vi "build.vi"(8 "error in (no error)":errorcluster, 10 "build_spec":T1, 11 "lv-build-default in":refnum<class "lv-builder.lvclass">) -> (0 "error out":errorcluster, 2 "[] generated_files":path[](array[path]), 3 "lv-build-default out":refnum<class "lv-builder.lvclass">)   [LabVIEW 2015, in "lv-builder.lvlib" / "lv-builder.lvclass"]
uses:
  lv-builder.lvclass
  lv-build/public/_controls/build_specification.ctl
  lv-build/public/_controls/build_type.ctl
  lv-builder.lvclass/lv-builder.ctl
  <vilib>/AppBuilder/AB_API_Simple/Set Build Specification Version (path).vi
  lv-builder.lvlib
  <vilib>/AppBuilder/AB_API_Simple/NI_App_Builder_API.lvlib
  lv-build/lv-build.lvlib
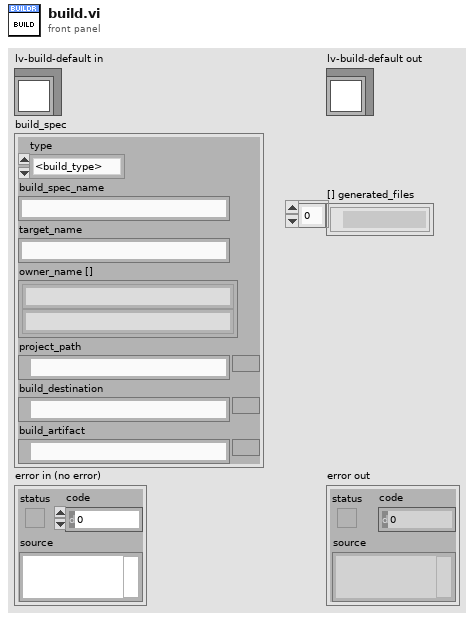
[diagram p1: front panel]
types:
  T1 = typedef "lv-build.lvlib/build_specification.ctl" = cluster{"type":T2, "build_spec_name":string, "target_name":string, "owner_name []":string[], "project_path":path, "build_destination":path, "build_artifact":path}
  T2 = typedef "lv-build.lvlib/build_type.ctl" = enum16{"<build_type>", "application_pc", "application_rt", "installer", "llb", "lvlibp", "zip", "fpga", "<null>"}
  T3 = typedef "NI_App_Builder_API.lvlib/Build Specification Version.ctl" = cluster{"Major":u16, "Minor":u16, "Fix":u16, "Build":u16}
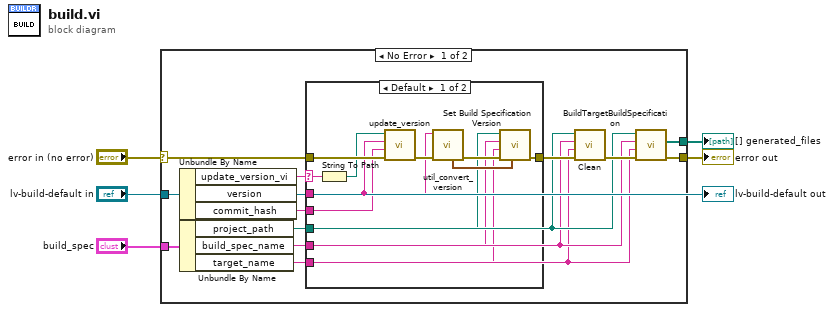
[diagram p0: block diagram]
diagram:
  n1 = case shown="No Error" "error in (no error)" {
    selector: "error in (no error)" -> [w16 w32]
    tunnel: [w10 w32] -> w3
    tunnel: "lv-build-default in" -> [w17 _]
    tunnel: "build_spec" -> [w18 _]
    tunnel: [w9 _] -> w2
    frame No Error {
      n2 = Unbundle By Name(w17) -> ("update_version_vi"=w15:string, "version"=w14:string, "commit_hash"=w13:string)
      n3 = Unbundle By Name(w18) -> ("project_path"=w8:path, "build_spec_name"=w7:string, "target_name"=w6:string)
      n4 = case shown="Default" w15 {
        selector: w15 -> [w28 _]
        tunnel: [w22 w31] -> w12
        tunnel: w14 -> [w25 _]
        tunnel: w13 -> [w26 _]
        tunnel: w16 -> [w29 w31]
        tunnel: w8 -> [w21 _]
        tunnel: w7 -> [w20 _]
        tunnel: w6 -> [w19 _]
        frame Default {
          n5 = String To Path(string=w28) -> (path=w27:path)
          n6 = call "update_version.vi"("error in (no error)"=w29, "commit_hash"=w26, "version"=w25, "version_vi"=w27) -> ("error out"=w30:errorcluster)  [unwired: 7 in]
          n7 = call "util_convert_version.vi"("error in (no error)"=w30, "version"=w25) -> ("error out"=w23:errorcluster, "build_specification_version"=w24:T3)  [unwired: 8 in]
          n8 = call-poly <vilib>:"Set Build Specification Version.vi"("Build Specification Version"=w24, "error in (no error)"=w23, "Name of target (My Computer)"=w19, "Name of build specification"=w20, "Path to project"=w21) -> ("error out"=w22:errorcluster)  [unwired: 6 in]
        }
        frame "" {
        }
      }
      n9 = call <vilib>:"Clean.vi"("error in (no error)"=w12, "Name of target (My Computer)"=w6, "Name of build specification (if empty: clean all)"=w7, "Path to project"=w8) -> ("error out"=w11:errorcluster)  [unwired: 7 in]
      n10 = call <vilib>:"BuildTargetBuildSpecification.vi"("error in (no error)"=w11, "Name of target (My Computer)"=w6, "Name of build specification (if empty: build all)"=w7, "Path to project"=w8) -> ("error out"=w10:errorcluster, "Generated files"=w9:path[])  [unwired: 6 in]
    }
    frame Error {
    }
  }
  "error out" <- w3
  "[] generated_files" <- w2
  "lv-build-default out" <- "lv-build-default in"
